vi "OASIS Image.vi"(6 "Path to Image\n(Empty - Use Picture)":path, 7 "Temp Path":path, 8 "Class (\"\")":string, 9 "Image Size (0,0)":cluster{"width":i32, "height":i32}, 10 "Image (Empty Picture)":picture, 11 "Previous HTML in":string) -> (0 "temp image file":path, 3 "HTML out":string)   [LabVIEW 2011]
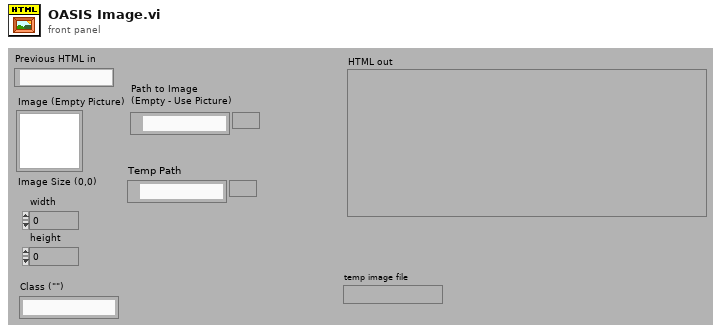
[diagram p1: front panel]
types:
  T1 = cluster{"left":i16, "top":i16, "right":i16, "bottom":i16}
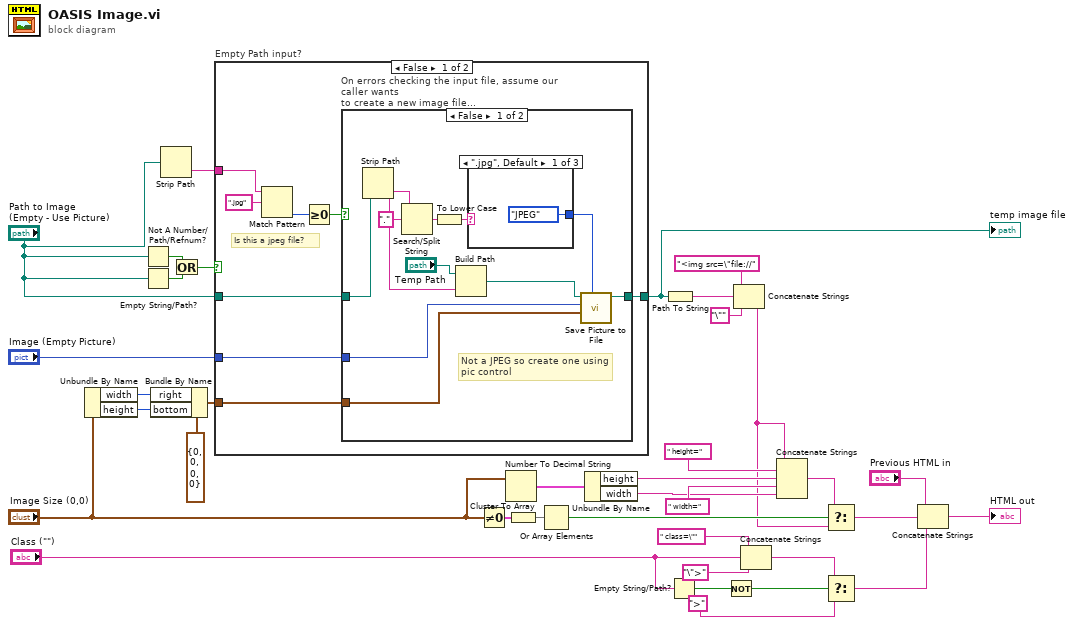
[diagram p0: block diagram]
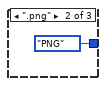
[diagram p2: hidden frame]
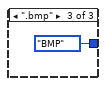
[diagram p3: hidden frame]
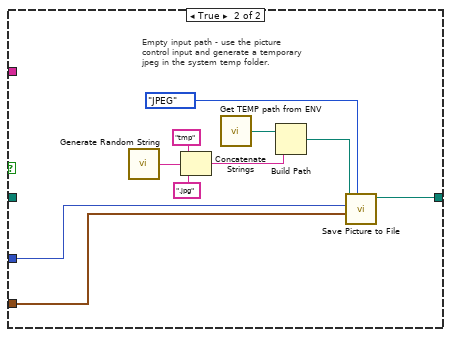
[diagram p5: hidden frame]
diagram:
  n1 = Unbundle By Name("Image Size (0,0)") -> ("width"=w6:i32, "height"=w7:i32)
  n2 = Not A Number/Path/Refnum?(number/path/refnum="Path to Image\n(Empty - Use Picture)") -> (NaN/Path/Refnum?=w10:bool)
  n3 = Empty String/Path?(string/path="Path to Image\n(Empty - Use Picture)") -> (empty?=w11:bool)
  n4 = Bundle By Name(cluster=T1 {"left"=0, "top"=0, "right"=0, "bottom"=0} ("rect"), "right"=w6, "bottom"=w7) -> (w3:T1)
  n5 = Strip Path(path="Path to Image\n(Empty - Use Picture)") -> (name=w1:string)  [unwired: 1 out]
  n6 = Or(x=w10, y=w11) -> (x .or. y?=w9:bool)
  n7 = case "Empty Path input?" shown="False" w9 {
    tunnel: [w44 w68] -> w13
    tunnel: "Path to Image\n(Empty - Use Picture)" -> [w41 _]
    tunnel: "Image (Empty Picture)" -> [w43 w66]
    tunnel: w3 -> [w42 w64]
    tunnel: w1 -> [w40 _]
    frame False {
      # "Is this a jpeg file?"
      n8 = Match Pattern(string=w40, regular expression=".jpg") -> (offset past match=w38:i32)  [unwired: 4 out]
      n9 = Greater Or Equal To 0?(x=w38) -> (x >= 0?=w37:bool)
      n10 = case "On errors checking the input file, assume our caller wants\nto create a new image file..." shown="False" w37 {
        tunnel: w41 -> [w51 w59]
        tunnel: [w54 w59] -> w44
        tunnel: w43 -> [w55 _]
        tunnel: w42 -> [w52 _]
        frame False {
          # "Not a JPEG so create one using\npic control"
          n11 = Strip Path(path=w51) -> (name=w46:string)  [unwired: 1 out]
          n12 = Search/Split String(string=w46, search string/char (-)=".") -> (match + rest of string=w49:string)  [unwired: 3 out]
          n13 = To Lower Case(string=w49) -> (all lower case string=w48:string)
          n14 = Build Path(base path="Temp Path", name or relative path=w46) -> (appended path=w47:path)
          n15 = case shown="\".jpg\", Default" w48 {
            tunnel: [enum16{"JPEG", "PNG", "BMP"}."JPEG" ("Image Format") enum16{"JPEG", "PNG", "BMP"}."PNG" ("Image Format") enum16{"JPEG", "PNG", "BMP"}."BMP" ("Image Format")] -> w53
            frame ".jpg", Default {
            }
            frame ".png" {
            }
            frame ".bmp" {
            }
          }
          n16 = call "Save Picture to File.vi"("Image Format"=w53, "rect"=w52, "Image (Empty Picture)"=w55, "path (empty prompts)"=w47) -> ("path out"=w54:path)  [unwired: 3 in, 4 out]
        }
        frame True {
          # "A valid JPEG path was given for\nthe img src.  Use that and ignore\nthe Picture input."
        }
      }
    }
    frame True {
      # "Empty input path - use the picture\ncontrol input and generate a temporary\njpeg in the system temp folder."
      n17 = call "Generate Random String.vi"() -> ("Output String"=w63:string)  [unwired: 1 in, 4 out]
      n18 = Concatenate Strings("tmp", w63, ".jpg") -> (w60:string)
      n19 = call "Get TEMP path from ENV.vi"() -> ("TEMP Path"=w69:path)  [unwired: 5 out]
      n20 = Build Path(base path=w69, name or relative path=w60) -> (appended path=w67:path)
      n21 = call "Save Picture to File.vi"("Image Format"=enum16{"JPEG", "PNG", "BMP"}."JPEG", "rect"=w64, "Image (Empty Picture)"=w66, "path (empty prompts)"=w67) -> ("path out"=w68:path)  [unwired: 3 in, 4 out]
    }
  }
  "temp image file" <- w13
  n22 = Not Equal To 0?(x="Image Size (0,0)") -> (x != 0?=w30:cluster{"width":bool, "height":bool})
  n23 = Number To Decimal String(number="Image Size (0,0)") -> (decimal integer string=w36:cluster{"width":string, "height":string})  [unwired: 1 out]
  n24 = Cluster To Array(cluster=w30) -> (array=w29:bool[])
  n25 = Or Array Elements(Boolean array=w29) -> (logical OR=w28:bool)
  n26 = Unbundle By Name(w36) -> ("height"=w35:string, "width"=w32:string)
  n27 = Path To String(path=w13) -> (string=w12:string)
  n28 = Empty String/Path?(string/path="Class (\"\")") -> (empty?=w25:bool)
  n29 = Not(x=w25) -> (.not. x?=w21:bool)
  n30 = Concatenate Strings("<img src=\"file://", w12, "\"") -> (w15:string)
  n31 = Concatenate Strings(" class=\"", "Class (\"\")", "\">") -> (w23:string)
  n32 = Concatenate Strings(w15, " height=", w35, " width=", w32) -> (w27:string)
  n33 = Select(t=w27, s=w28, f=w15) -> (s? t:f=w18:string)
  n34 = Select(t=w23, s=w21, f=">") -> (s? t:f=w14:string)
  n35 = Concatenate Strings("Previous HTML in", w18, w14) -> (→"HTML out":string)
